vi "process_KEITHLEY_2260B.vi"(3 "Cluster":T1={"COM PORT"="COM9", "cmd"="*IDN?", "type"="write_and_read", "delay"="100", "格式"="asc,search", "min"="2260B", "max"="", "備註"="qqqqq"}) -> (0 "error out":errorcluster, 1 "2260B_output":string[](array[string]))   [LabVIEW 2026]
uses:
  <vilib>/Instr/_visa.llb/VISA Configure Serial Port (Instr).vi
panel:
  out "read buffer":string
  in  "2260 COM PORT":refnum<visa-resource-name>
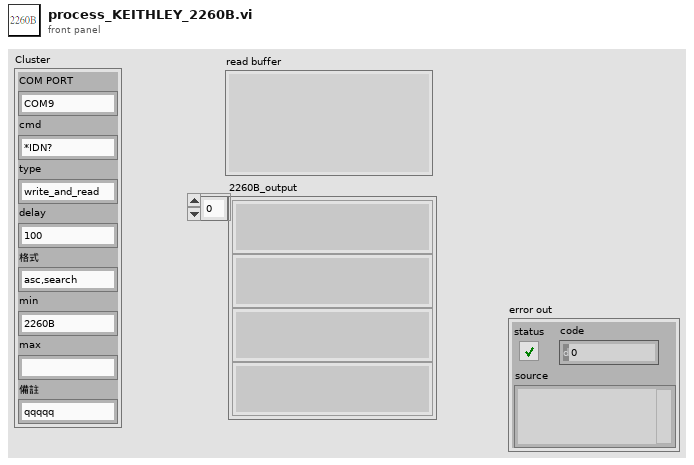
[diagram p1: front panel]
types:
  T1 = cluster{"COM PORT":string, "cmd":string, "type":string, "delay":string, "格式":string, "min":string, "max":string, "備註":string}
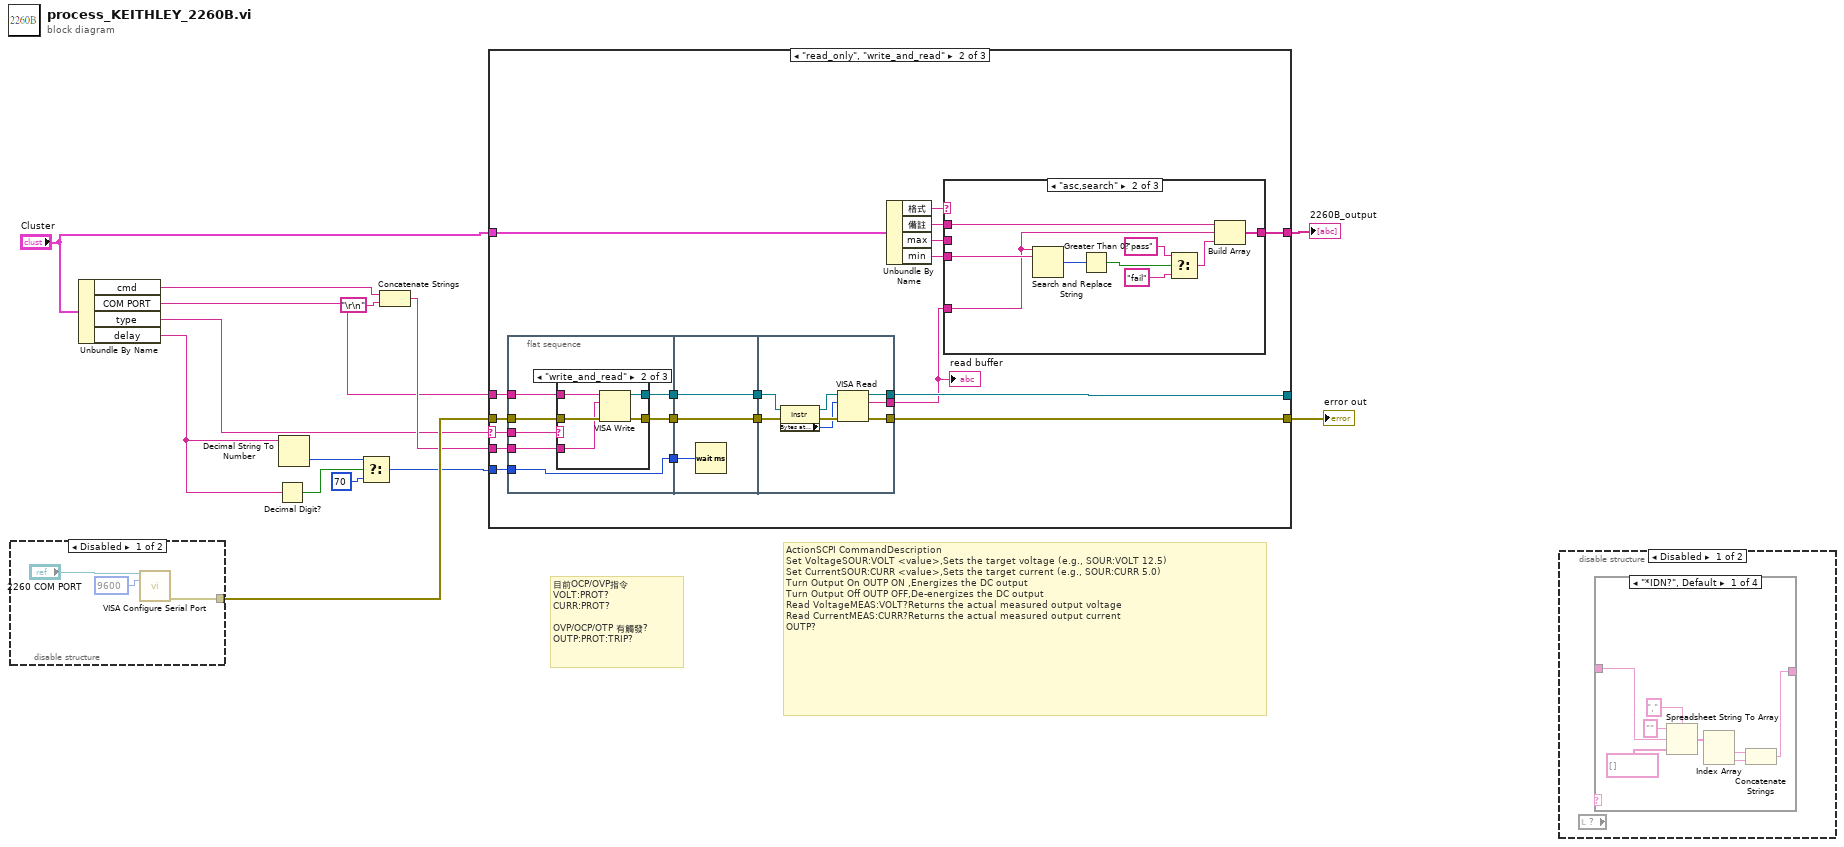
[diagram p0: block diagram]
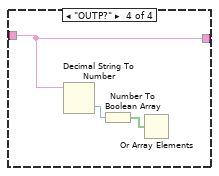
[diagram p5: hidden frame]
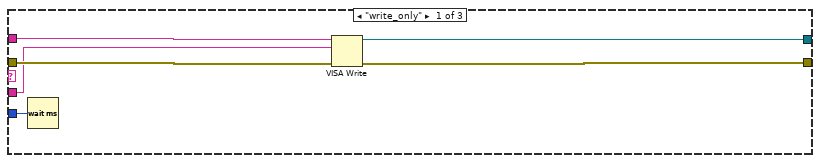
[diagram p7: hidden frame]
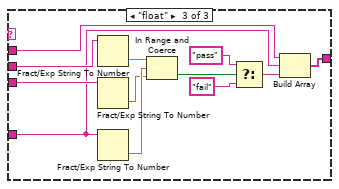
[diagram p9: hidden frame]
diagram:
  # "目前OCP/OVP指令\nVOLT:PROT?\nCURR:PROT?\n\nOVP/OCP/OTP 有觸發?\nOUTP:PROT:TRIP?"
  # "ActionSCPI CommandDescription\nSet VoltageSOUR:VOLT <value>,Sets the target voltage (e.g., SOUR:VOLT 12.5)\nSet CurrentSOUR:CURR <value>,Sets the target current (e.g., SOUR:CURR 5.0)\nTurn Output On OUTP ON ,Energizes the DC output\nTurn Output Off OUTP OFF,De-energizes the DC output\nRead VoltageMEAS:VOLT?Returns the actual measured output voltage\nRead CurrentMEAS:CURR?Returns the actual measured output current\nOUTP?"
  n1 = disable-structure shown="Disabled" {
    disable-tunnel: [w15 _] -> w13
    frame Disabled {
      n2 = call-poly "VISA Configure Serial Port"("VISA resource name"="2260 COM PORT", "baud rate (9600)"=u32 9600) -> ("error out"=w15:errorcluster)  [unwired: 12 in, 1 out]
    }
    frame Enabled {
    }
  }
  n3 = Unbundle By Name("Cluster") -> ("cmd"=w4:string, "COM PORT"=w2:string, "type"=w5:string, "delay"=w3:string)
  n4 = Decimal Digit?(1:w3) -> (0:w10:bool)
  n5 = Decimal String To Number(string=w3) -> (number=w8:i32)  [unwired: 2 in, 1 out]
  n6 = Select(t=w8, s=w10, f=u32 70 ("milliseconds to wait")) -> (s? t:f=w6:u32)
  n7 = Concatenate Strings(w4, "\r\n") -> (w12:string)
  n8 = case shown="\"read_only\", \"write_and_read\"" w5 {
    selector: w5 -> [_ w24 _]
    tunnel: w2 -> [w23 w42 w92]
    tunnel: w13 -> [w22 w41 w91]
    tunnel: w12 -> [w21 w32 _]
    tunnel: w6 -> [w20 w39 _]
    tunnel: [w19 w34 w92] -> _
    tunnel: [w18 w33 w91] -> w1
    tunnel: [_ w31 _] -> w11
    tunnel: "Cluster" -> [_ w29 _]
    frame "write_only" {
      n9 = Wait (ms)(milliseconds to wait=w20) -> ()  [unwired: 1 out]
      n10 = VISA Write(VISA resource name=w23, write buffer=w21, error in (no error)=w22) -> (VISA resource name out=w19:refnum<visa-resource-name>, error out=w18:errorcluster)  [unwired: 1 out]
    }
    frame "read_only", "write_and_read" {
      n11 = flat-sequence {
        tunnel: w42 -> [w66]
        tunnel: w41 -> [w68]
        tunnel: [w70] -> w40
        tunnel: w39 -> [w70]
        tunnel: [w64] -> w38
        tunnel: [w65] -> w35
        tunnel: w32 -> [w67]
        tunnel: w24 -> [w69]
        tunnel: w40 -> [w80]
        tunnel: w38 -> [w82]
        tunnel: [w82] -> w37
        tunnel: [w81] -> w36
        tunnel: w35 -> [w81]
        tunnel: w37 -> [w87]
        tunnel: w36 -> [w86]
        tunnel: [w85] -> w30
        tunnel: [w84] -> w34
        tunnel: [w83] -> w33
        frame #0 {
          n12 = case shown="\"write_and_read\"" w69 {
            tunnel: w68 -> [w71 w77 w78]
            tunnel: w67 -> [_ w76 _]
            tunnel: w66 -> [w72 w75 w79]
            tunnel: [w71 w74 w78] -> w65
            tunnel: [w72 w73 w79] -> w64
            frame "", Default {
            }
            frame "write_and_read" {
              n13 = VISA Write(VISA resource name=w75, write buffer=w76, error in (no error)=w77) -> (VISA resource name out=w73:refnum<visa-resource-name>, error out=w74:errorcluster)  [unwired: 1 out]
            }
            frame "read_only" {
            }
          }
        }
        frame #1 {
          n14 = Wait (ms)(milliseconds to wait=w80) -> ()  [unwired: 1 out]
        }
        frame #2 {
          n15 = property class="Instr"(reference=w87, error in=w86) -> (reference out=w88:refnum<visa-resource-name>, error out=w90:errorcluster, "Bytes at Port"=w89:u32)
          n16 = VISA Read(VISA resource name=w88, byte count=w89, error in (no error)=w90) -> (VISA resource name out=w84:refnum<visa-resource-name>, read buffer=w85:string, error out=w83:errorcluster)  [unwired: 1 out]
        }
      }
      n17 = Unbundle By Name(w29) -> ("格式"=w27:string, "備註"=w28:string, "max"=w26:string, "min"=w25:string)
      n18 = case shown="\"asc,search\"" w27 {
        tunnel: w25 -> [_ w44 w53]
        tunnel: w28 -> [_ w50 w63]
        tunnel: w26 -> [_ _ w62]
        tunnel: [_ w45 w54] -> w31
        tunnel: w30 -> [_ w43 w52]
        frame "False", Default {
        }
        frame "asc,search" {
          n19 = Search and Replace String(input string=w43, search string=w44) -> (number of replacements=w51:i32)  [unwired: 6 in, 3 out]
          n20 = Greater Than 0?(x=w51) -> (x > 0?=w46:bool)
          n21 = Select(t="pass", s=w46, f="fail") -> (s? t:f=w48:string)
          n22 = Build Array(w50, w43, w48) -> (w45:string[])
        }
        frame "float" {
          n23 = Fract/Exp String To Number(string=w62) -> (number=w59:dbl)  [unwired: 3 in, 1 out]
          n24 = Fract/Exp String To Number(string=w53) -> (number=w60:dbl)  [unwired: 3 in, 1 out]
          n25 = Fract/Exp String To Number(string=w52) -> (number=w61:dbl)  [unwired: 3 in, 1 out]
          n26 = In Range and Coerce(upper limit=w59, x=w61, lower limit=w60) -> (In Range?=w55:bool)  [unwired: 1 out]
          n27 = Select(t="pass", s=w55, f="fail") -> (s? t:f=w56:string)
          n28 = Build Array(w63, w52, w56) -> (w54:string[])
        }
      }
      "read buffer" <- w30
    }
    frame "", Default {
    }
  }
  "error out" <- w1
  "2260B_output" <- w11
  n29 = disable-structure shown="Disabled" {
    frame Disabled {
      n30 = local read item#-1() -> ()  [unwired: 1 out]
      n31 = case shown="\"*IDN?\", Default" w93 {
        tunnel: _ -> [w95 w102 w103 w104]
        tunnel: [w94 w102 w103 w104] -> _
        frame "*IDN?", Default {
          n32 = Spreadsheet String To Array(delimiter (Tab)="," ("format string"), format string="", spreadsheet string=w95, array type (2D Dbl)=string[] []) -> (array=w99:string[])
          n33 = Index Array(array=w99) -> (element #1=w100:string, element #2=w101:string)  [unwired: 2 in]
          n34 = Concatenate Strings(w100, w101) -> (w94:string)
        }
        frame "MEAS:VOLT?" {
        }
        frame "MEAS:CURR?" {
        }
        frame "OUTP?" {
          n35 = Decimal String To Number(string=w104) -> (number=w106:i32)  [unwired: 2 in, 1 out]
          n36 = Number To Boolean Array(number=w106) -> (Boolean array=w105:bool[])
          n37 = Or Array Elements(Boolean array=w105) -> ()  [unwired: 1 out]
        }
      }
    }
    frame Enabled {
    }
  }
